vi "PXI-Write DO Buffers.vi"(0 "DO Tasks":T1[](array[typedef]), 2 "zero output":bool, 7 "DO Waveforms":bool[][](array[boolean]), 11 "error in (no error)":errorcluster, 12 "Force write":bool) -> (4 "DO Tasks out":T1[](array[typedef]), 15 "error out":errorcluster)   [LabVIEW 2020]
uses:
  Type Defs/Task Struct.ctl
  <vilib>/DAQmx/write.llb/DAQmx Write (Digital Wfm 1Chan NSamp).vi
  <vilib>/Waveform/DWDTOps.llb/DWDT Boolean Array to Digital.vi
  <vilib>/Waveform/DWDTOps.llb/DWDT Uncompress Digital.vi
  <vilib>/DAQmx/miscellaneous.llb/DAQmx Fill In Error Info.vi
  <resource>/objmgr/daqmx.rc
panel:
  out "Waveform Graph":i16[][](graph)
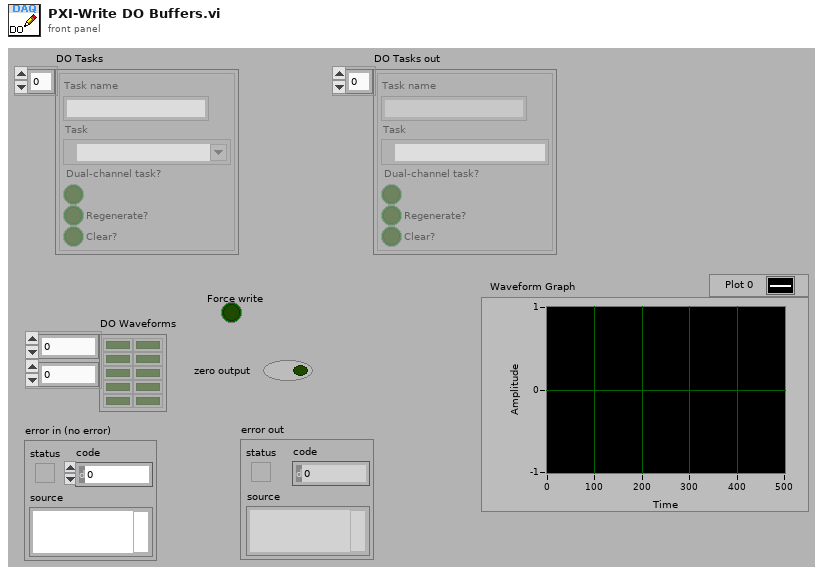
[diagram p1: front panel]
types:
  T1 = typedef "Task Struct.ctl" = cluster{"Task name":string, "Task":refnum<k21>, "Dual-channel task?":bool, "Regenerate?":bool, "Clear?":bool}
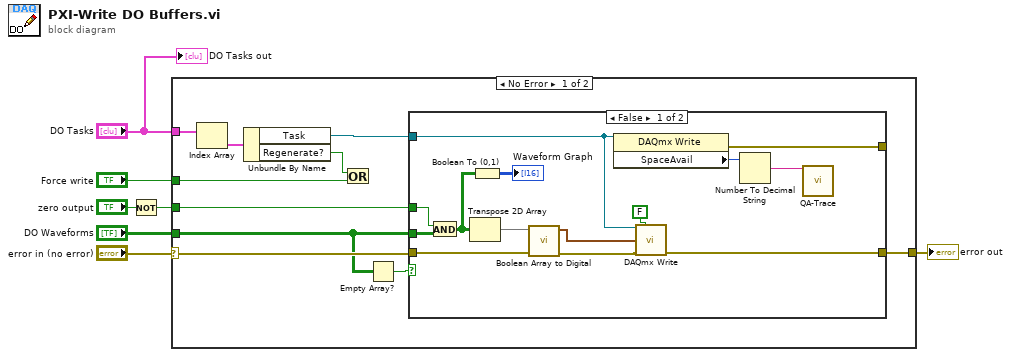
[diagram p0: block diagram]
diagram:
  n1 = Not(x="zero output") -> (.not. x?=w4:bool)
  n2 = case shown="No Error" "error in (no error)" {
    selector: "error in (no error)" -> [w12 w33]
    tunnel: [w17 w33] -> w7
    tunnel: "DO Tasks" -> [w16 _]
    tunnel: "DO Waveforms" -> [w8 _]
    tunnel: w4 -> [w10 _]
    tunnel: "Force write" -> [w11 _]
    frame No Error {
      n3 = Index Array(array=w16) -> (element=w15:T1)  [unwired: 1 in]
      n4 = Unbundle By Name(w15) -> ("Task"=w14:refnum<k21>, "Regenerate?"=w13:bool)
      n5 = Or(x=w13, y=w11) -> ()  [unwired: 1 out]
      n6 = Empty Array?(array=w8) -> (empty?=w9:bool)
      n7 = case shown="False" w9 {
        tunnel: w14 -> [w21 _]
        tunnel: w12 -> [w29 w32]
        tunnel: [w22 w32] -> w17
        tunnel: w8 -> [w31 _]
        tunnel: w10 -> [w30 _]
        tunnel: [w18 _] -> _
        frame False {
          n8 = And(x=w30, y=w31) -> (x .and. y?=w23:bool[][])
          n9 = Transpose 2D Array(2D array=w23) -> (transposed array=w25:bool[][])
          n10 = Boolean To (0,1)(Boolean=w23) -> (0, 1=→"Waveform Graph":i16[][])
          n11 = call-poly <vilib>:"Boolean Array to Digital.vi"("error in (no error)"=w29, "boolean array"=w25) -> ("error out"=w28:errorcluster, "digital waveform"=w26:digitalwaveform)  [unwired: 8 in]
          n12 = property class="DAQmx Write"(reference=w21) -> (error out=w18:errorcluster, "SpaceAvail"=w20:u32)  [unwired: 1 in, 1 out]
          n13 = call-poly <vilib>:"DAQmx Write.vi"("task/channels in"=w21, "auto start"=FALSE, "data"=w26, "error in"=w28) -> ("error out"=w22:errorcluster)  [unwired: 9 in, 2 out]
          n14 = Number To Decimal String(number=w20) -> (decimal integer string=w19:string)  [unwired: 1 in]
          n15 = call "QA-Trace.vi"("trace string"=w19) -> ()  [unwired: 14 in, 1 out]
        }
        frame True {
        }
      }
    }
    frame Error {
    }
  }
  "error out" <- w7
  "DO Tasks out" <- "DO Tasks"
